vi "Serialize.vi"(8 "error in (no error)":errorcluster, 10 "Item Info":refnum<class "XML Node.lvclass">, 11 "ZIP Item in":refnum<class "ZIP Item.lvclass">) -> (0 "error out":errorcluster, 2 "Serialization Version":string)   [LabVIEW 2019, in "ZIP.lvlib" / "ZIP Item.lvclass"]
uses:
  ZIP Item.lvclass
  libs/Solution.lvlibp/Solution/XML Reader/XML Node.lvclass
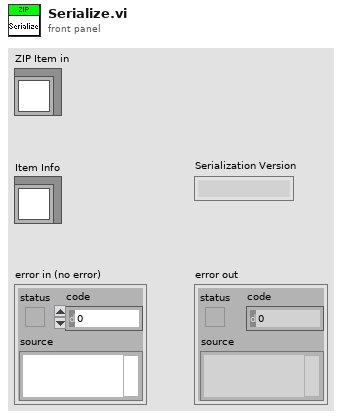
[diagram p1: front panel]
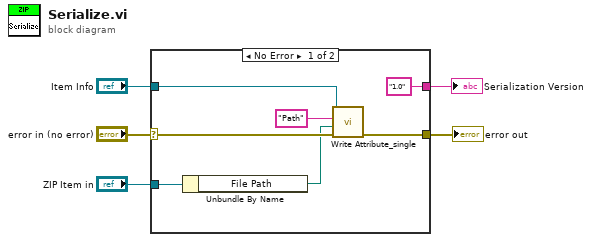
[diagram p0: block diagram]
diagram:
  n1 = case shown="No Error" "error in (no error)" {
    selector: "error in (no error)" -> [w12 w13]
    tunnel: [w11 w13] -> w4
    tunnel: "Item Info" -> [w10 _]
    tunnel: "ZIP Item in" -> [w8 _]
    tunnel: ["1.0" _] -> w1
    frame No Error {
      n2 = Unbundle By Name(w8) -> ("File Path"=w7:path)
      n3 = call "Write Attribute_single.vi"("error in (no error)"=w12, "Value"=w7, "Name"="Path", "XML Node in"=w10) -> ("error out"=w11:errorcluster)  [unwired: 7 in]
    }
    frame Error {
    }
  }
  "error out" <- w4
  "Serialization Version" <- w1
